vi "Write Signals Refnum.vi"(8 "error in (no error)":errorcluster, 10 "Signals Refnum":refnum<vi>, 11 "Universal Display in":refnum<class "Universal Display.lvclass">) -> (0 "error out":errorcluster, 3 "Universal Display out":refnum<class "Universal Display.lvclass">)   [LabVIEW 2016, in "Display Panel.lvlib" / "Universal Display.lvclass"]
uses:
  Universal Display.lvclass
  Universal Display.lvclass/Universal Display.ctl
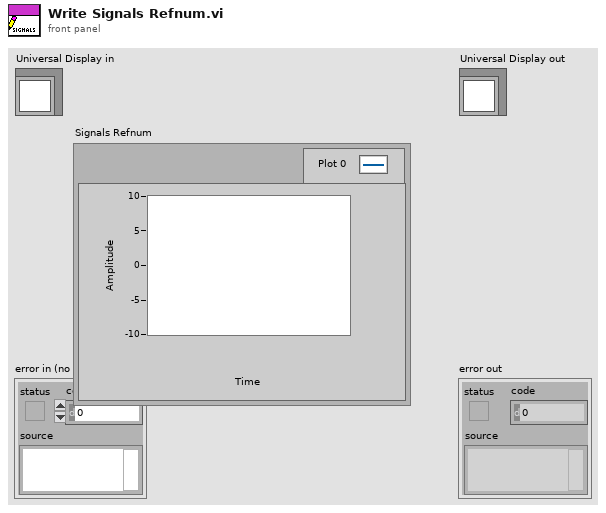
[diagram p1: front panel]
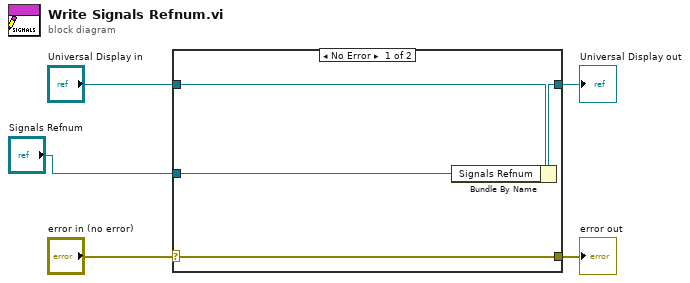
[diagram p0: block diagram]
diagram:
  n1 = case shown="No Error" "error in (no error)" {
    selector: "error in (no error)" -> [w9 w10]
    tunnel: [w9 w10] -> w4
    tunnel: [w7 w11] -> w2
    tunnel: "Universal Display in" -> [w8 w11]
    tunnel: "Signals Refnum" -> [w6 _]
    frame No Error {
      n2 = Bundle By Name(cluster=w8, "Signals Refnum"=w6) -> (w7:refnum<class "Universal Display.lvclass">)
    }
    frame Error {
    }
  }
  "error out" <- w4
  "Universal Display out" <- w2
